vi "Close Device.vi"(8 "error in (no error)":errorcluster, 11 "Simulated Waveform in":refnum<class "Simulated Waveform.lvclass">) -> (0 "error out":errorcluster, 3 "Simulated Waveform out":refnum<class "Simulated Waveform.lvclass">)   [LabVIEW 2020, in "Simulated Waveform.lvlib" / "Simulated Waveform.lvclass"]
uses:
  Simulated Waveform.lvclass
  Simulated Waveform.lvclass/Simulated Waveform.ctl
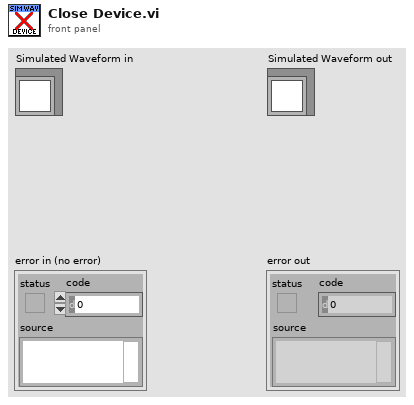
[diagram p1: front panel]
types:
  T1 = typedef "Simulated Waveform.lvlib/Simulated Waveform.lvclass/Ref Data.ctl" = cluster{"Sim Queue Name":string, "Waveform Queue":refnum<queue>, "Noise Factor":dbl}
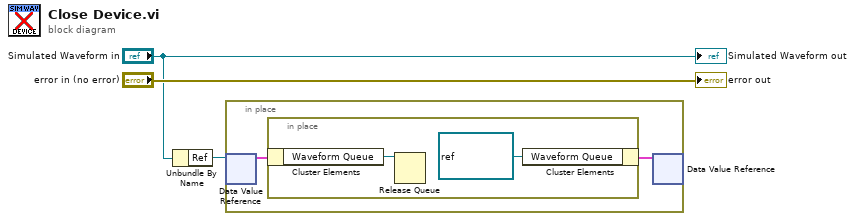
[diagram p0: block diagram]
diagram:
  n1 = Unbundle By Name("Simulated Waveform in") -> ("Ref"=w2:refnum<data-value>)
  n2 = in-place {
    n3 = in-place-dvr #1(w2) -> (w5:T1)  [unwired: 1 out]
    n4 = in-place {
      n5 = in-place-cluster #2(w5) -> ("Waveform Queue"=w7:refnum<queue>)
      n6 = Release Queue(queue=w7) -> ()  [unwired: 2 in, 3 out]
      n7 = in-place-cluster #2("Waveform Queue"=refnum<queue> refnum) -> (w4:T1)
    }
    n8 = in-place-dvr #1(w4) -> ()  [unwired: 2 out]
  }
  "error out" <- "error in (no error)"
  "Simulated Waveform out" <- "Simulated Waveform in"
